vi "fpga_Freq Lowpass filter (P Class_50Hz).vi"(0 "input data":fxp<+/-,24,2>, 1 "reset":bool, 9 "input valid":bool) -> (4 "output data":fxp<+/-,24,3>, 10 "output valid":bool, 14 "ready for input":bool)   [LabVIEW 2013, in "NI_EP_PMU_FPGA.lvlib"]
doc: "----------------------\n\nThis filter is configured as follows:\n\n<b>Filter Configuration</b>\nType: Single Rate\nStructure: FIR Direct Form\n\n<b>Input Data Type</b>\nType: fixed-point <±,24,2> [-2.000000E+0,2.000000E+0]:2.384186E-7\n\n<b>Output Data Type</b>\nType: fixed-point <±,24,3> [-4.000000E+0,4.000000E+0]:4.768372E-7\nRounding mode: Truncate\nOverflow mode: Wrap\n\n<b>Implementation</b>\nNumber of channels: 1\nMaximum input sampling rate per channel @ 40MHz: 1.026MHz\nGain processing: On Host\nMethod: Multiply-Accumulate\nNumber of multiply pipeline stages: 1\nMultiply register in: False\nNumber of adder levels per register: 2\nState memory: Look-Up Table\nCoefficient memory: ROM\n\n<b>Execution Mode</b>\nInside single-cycle Timed Loop\nThroughput: 39 cycles/sample\n\n<b>Estimated Resources</b>\nNumber of multiply-accumulate units: 1\nMultiply operation: I24.2 x I16.-2 => I40.3"
uses:
  <vilib>/addons/Electrical Power/PMU/NI_EP_PMU_FPGA.lvlib
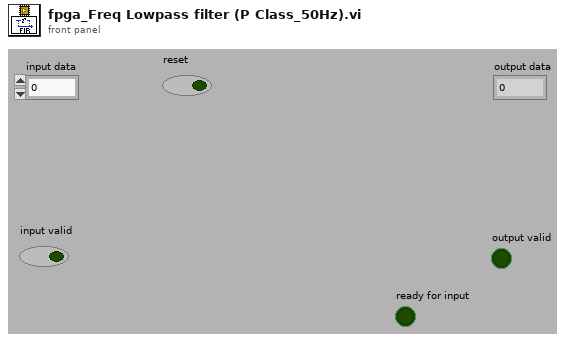
[diagram p1: front panel]
types:
  T1 = cluster{"WREn":bool, "WRAddr":fxp<+,6,6>, "RDAddr":fxp<+,6,6>, "BufWREn":bool, "BufWRAddr":fxp<+,6,6>, "firstRun":bool, "BufFiirstRun":bool}
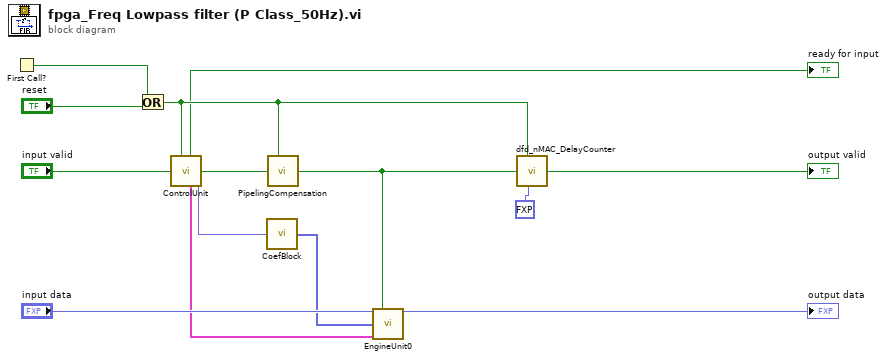
[diagram p0: block diagram]
diagram:
  n1 = First Call?() -> (First Call?: T/F=w11:bool)
  n2 = Or(x=w11, y="reset") -> (x .or. y?=w10:bool)
  n3 = call "ControlUnit"("reset"=w10, "input valid"="input valid") -> ("ready for input"=→"ready for input":bool, "output valid"=w13:bool, "opState"=w6:T1, "coefRDAddr"=w8:fxp<+,6,6>)  [unwired: 4 in]
  n4 = call "CoefBlock"("coefAddr"=w8) -> ("coefficients"=w2:fxp<+/-,16,-2>[])  [unwired: 8 in]
  n5 = call "PipelingCompensation"("reset"=w10, "data in"=w13) -> ("data out"=w5:bool)  [unwired: 7 in]
  n6 = call "EngineUnit0"("input data"="input data", "ACC_Load"=w5, "coefficients"=w2, "opState"=w6) -> ("output data"=→"output data":fxp<+/-,24,3>)  [unwired: 11 in]
  n7 = call "dfd_nMAC_DelayCounter.vi"("reset"=w10, "data in"=w5, "#delay"=fxp<+,6,6> 39.0 ("#TPPM")) -> ("data out"=→"output valid":bool)  [unwired: 6 in]
